vi "Farberkennung.vi"(8 "error in (no error)":errorcluster caption="Fehler (Eingang, kein Fehler)", 10 "Farbwerte":T2, 11 "Device ID":T1(ring)) -> (0 "error out":errorcluster caption="Fehler (Ausgang)", 1 "Fertig":bool, 2 "Farbe":u16(ring) items=["Blau", "Weiß", "Grün", "unknew", "Rot"], 3 "Device ID Out":T1(ring))   [LabVIEW 2010]
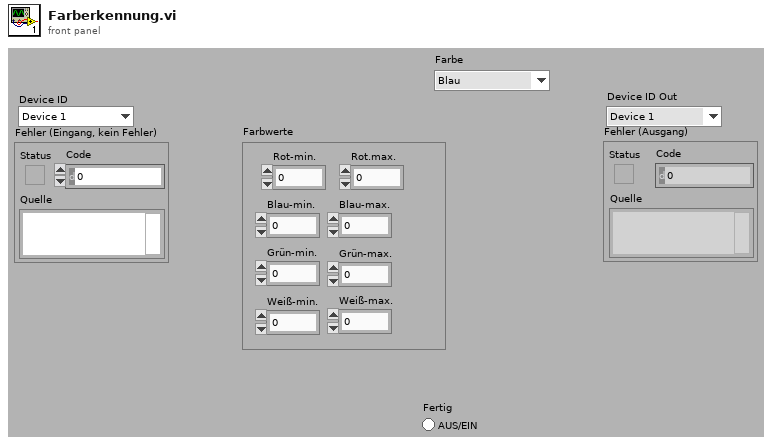
[diagram p1: front panel]
types:
  T1 = enum16{"Device 1", "Device 2", "Device 3", "Device 4", "Device 5", "Device 6", "Device 7", "Device 8"}
  T2 = cluster{"Rot-min.":dbl, "Rot.max.":dbl, "Blau-min.":dbl, "Blau-max.":dbl, "Grün-min.":dbl, "Grün-max.":dbl, "Weiß-min.":dbl, "Weiß-max.":dbl}
  T3 = enum8{"Input AX", "Input AY", "Input A1", "Input A2", "Input AZ", "Input AV", "Input D1", "Input D2", "Input AXR", "Input AYR"}
  T4 = enum8{"Robo Interface", "Extension 1", "Extension 2", "Extension 3"}
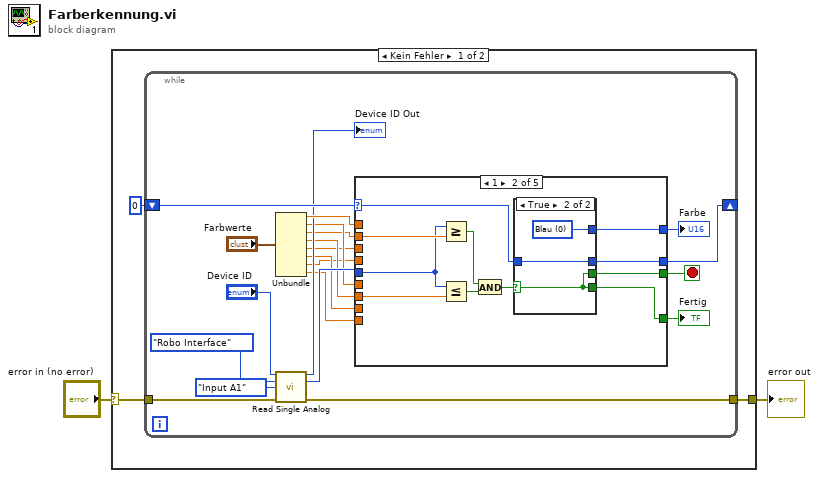
[diagram p0: block diagram]
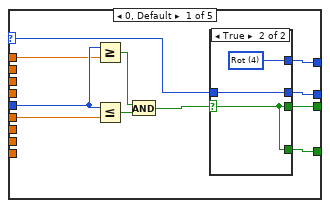
[diagram p2: hidden frame]
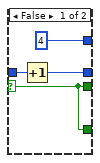
[diagram p3: hidden frame]
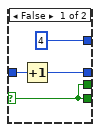
[diagram p4: hidden frame]
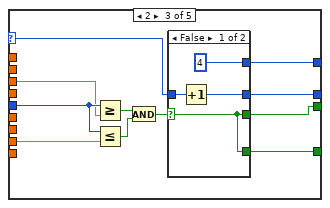
[diagram p5: hidden frame]
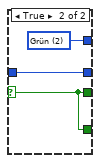
[diagram p6: hidden frame]
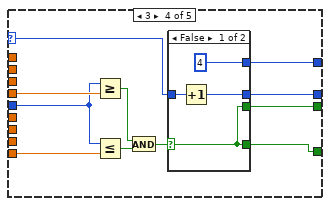
[diagram p7: hidden frame]
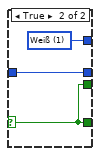
[diagram p8: hidden frame]
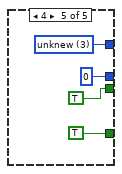
[diagram p9: hidden frame]
diagram:
  n1 = case shown="Kein Fehler" "error in (no error)" {
    selector: "error in (no error)" -> [w5 w103]
    tunnel: [w4 w103] -> w1
    frame No Error {
      n2 = while {
        tunnel: w5 -> [w25]
        tunnel: [w24] -> w4
        shift-right: [w22] -> _
        shift-left: 0 -> [w23]
        stop <- w17 stop-if-true
        n3 = Unbundle("Farbwerte") -> ("Rot-min."=w20:dbl, "Rot.max."=w15:dbl, "Blau-min."=w14:dbl, "Blau-max."=w13:dbl, "Grün-min."=w11:dbl, "Grün-max."=w10:dbl, "Weiß-min."=w9:dbl, "Weiß-max."=w8:dbl)
        n4 = call "Read Single Analog.vi"("Device ID"="Device ID", "Module"=T4."Robo Interface", "Analog_Input"=T3."Input A1", "error in"=w25) -> ("Device ID Out"=→"Device ID Out":T1, "Value"=w18:u16, "error out"=w24:errorcluster)  [unwired: 9 out]
        n5 = case shown="1" w23 {
          selector: w23 -> [w37 w51 w66 w84 _]
          tunnel: [w36 w48 w68 w86 0] -> w22
          tunnel: w20 -> [w34 _ _ _ _]
          tunnel: w18 -> [w35 w50 w65 w81 _]
          tunnel: [w30 w47 w69 w87 TRUE] -> w17
          tunnel: [w29 w49 w67 w85 w102] -> w16
          tunnel: w15 -> [w28 _ _ _ _]
          tunnel: w14 -> [_ w52 _ _ _]
          tunnel: w13 -> [_ w45 _ _ _]
          tunnel: [w27 w46 w70 w88 TRUE] -> w12
          tunnel: w11 -> [_ _ w64 _ _]
          tunnel: w10 -> [_ _ w63 _ _]
          tunnel: w9 -> [_ _ _ w83 _]
          tunnel: w8 -> [_ _ _ w82 _]
          frame 0, Default {
            n6 = Greater Or Equal? ("Größer oder gleich?")(x=w35, y=w34) -> (x >= y?=w32:bool)
            n7 = Less Or Equal? ("Kleiner oder gleich?")(x=w35, y=w28) -> (x <= y?=w33:bool)
            n8 = And(x=w32, y=w33) -> (x .and. y?=w31:bool)
            n9 = case shown="TRUE" w31 {
              selector: w31 -> [w38 w42]
              tunnel: w37 -> [w41 w44]
              tunnel: [w40 w44] -> w36
              tunnel: [w38 w42] -> w30
              tunnel: [u16 4 ("Farbe") w43] -> w29
              tunnel: [w38 w42] -> w27
              frame False {
                n10 = Increment(x=w41) -> (x+1=w40:i32)
              }
              frame True {
                w43 = u16 4 items=["Blau", "Weiß", "Grün", "unknew", "Rot"] ("Farbe")
              }
            }
          }
          frame 1 {
            n11 = Greater Or Equal?(x=w50, y=w52) -> (x >= y?=w54:bool)
            n12 = Less Or Equal?(x=w50, y=w45) -> (x <= y?=w55:bool)
            n13 = And(x=w54, y=w55) -> (x .and. y?=w53:bool)
            n14 = case shown="TRUE" w53 {
              selector: w53 -> [w56 w60]
              tunnel: w51 -> [w59 w62]
              tunnel: [w58 w62] -> w48
              tunnel: [w56 w60] -> w47
              tunnel: [u16 4 ("Farbe") w61] -> w49
              tunnel: [w56 w60] -> w46
              frame False {
                n15 = Increment(x=w59) -> (x+1=w58:i32)
              }
              frame True {
                w61 = u16 0 items=["Blau", "Weiß", "Grün", "unknew", "Rot"] ("Farbe")
              }
            }
          }
          frame 2 {
            n16 = Greater Or Equal?(x=w65, y=w64) -> (x >= y?=w72:bool)
            n17 = Less Or Equal?(x=w65, y=w63) -> (x <= y?=w73:bool)
            n18 = And(x=w72, y=w73) -> (x .and. y?=w71:bool)
            n19 = case shown="FALSE" w71 {
              selector: w71 -> [w74 w78]
              tunnel: w66 -> [w77 w80]
              tunnel: [w76 w80] -> w68
              tunnel: [w74 w78] -> w69
              tunnel: [u16 4 ("Farbe") w79] -> w67
              tunnel: [w74 w78] -> w70
              frame False {
                n20 = Increment(x=w77) -> (x+1=w76:i32)
              }
              frame True {
                w79 = u16 2 items=["Blau", "Weiß", "Grün", "unknew", "Rot"] ("Farbe")
              }
            }
          }
          frame 3 {
            n21 = Greater Or Equal?(x=w81, y=w83) -> (x >= y?=w90:bool)
            n22 = Less Or Equal?(x=w81, y=w82) -> (x <= y?=w91:bool)
            n23 = And(x=w90, y=w91) -> (x .and. y?=w89:bool)
            n24 = case shown="FALSE" w89 {
              selector: w89 -> [w92 w96]
              tunnel: w84 -> [w95 w98]
              tunnel: [w94 w98] -> w86
              tunnel: [w92 w96] -> w87
              tunnel: [u16 4 ("Farbe") w97] -> w85
              tunnel: [w92 w96] -> w88
              frame False {
                n25 = Increment(x=w95) -> (x+1=w94:i32)
              }
              frame True {
                w97 = u16 1 items=["Blau", "Weiß", "Grün", "unknew", "Rot"] ("Farbe")
              }
            }
          }
          frame 4 {
            w102 = u16 3 items=["Blau", "Weiß", "Grün", "unknew", "Rot"] ("Farbe")
          }
        }
        "Farbe" <- w16
        "Fertig" <- w12
      }
    }
    frame Error {
    }
  }
  "error out" <- w1
